vi "myVTOL Read-Write.vi"(5 "Fan Power Control (0V)":dbl(slide) scale=0.0..10.0, 7 "Control Mode (Manual)":bool, 8 "Error In":errorcluster, 9 "PID Settings":T1={"Proportional"=1.0, "Integral"=0.03, "Derivative"=0.05} {"Derivative" format="%.3f"; "Integral" format="%.2f"; "Proportional" format="%.3f"}, 10 "Set Point (2.1V)":dbl=2.1 step=0.01 format="%#_g V", 11 "task array in":refnum<k21>[](array[refnum])) -> (0 "Error Out":errorcluster, 1 "Sensor Reading":dbl=2.0424252344528213 format="%0.2f V", 2 "Fan Control Output [V]":dbl(knob)=5.428571428571428 scale=0.0..10.0, 3 "task array out":refnum<k21>[](array[refnum]), 4 "Waveform Chart":cluster{"data":dbl, "Set Point":dbl}(graph)={"data"=2.0424252344528213, "Set Point"=2.1})   [LabVIEW 2013]
uses:
  <vilib>/DAQmx/read.llb/DAQmx Read (Analog Wfm 1Chan NSamp).vi
  <vilib>/DAQmx/write.llb/DAQmx Write (Analog DBL 1Chan 1Samp).vi
  <vilib>/DAQmx/miscellaneous.llb/DAQmx Fill In Error Info.vi
panel:
  # "PID Gain Settings"
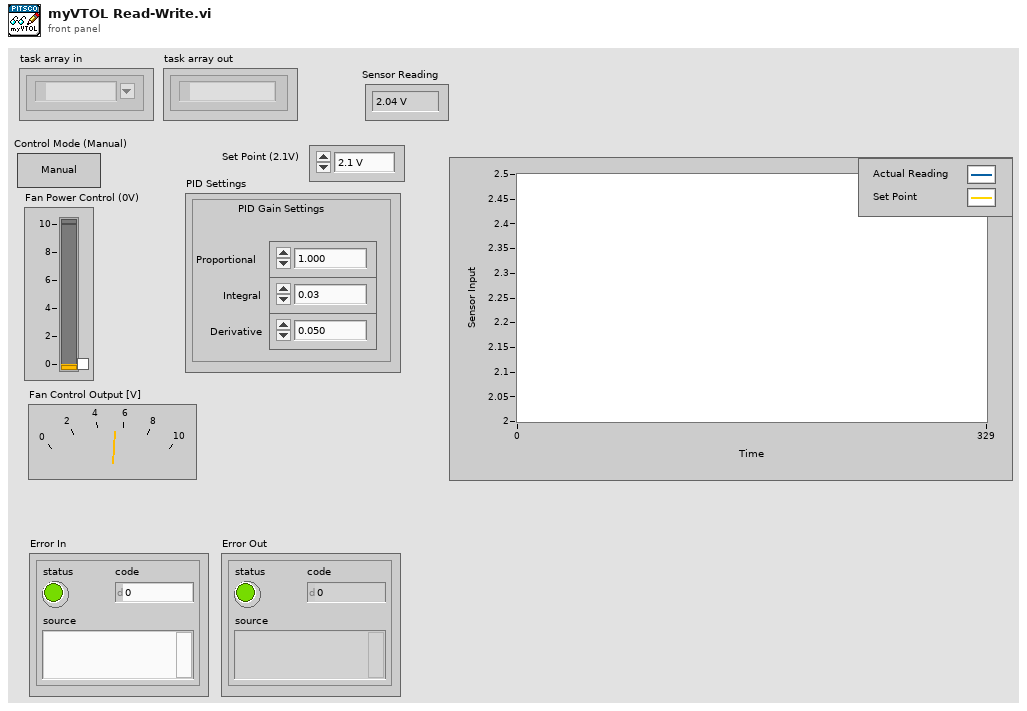
[diagram p1: front panel]
types:
  T1 = cluster{"Proportional":dbl, "Integral":dbl, "Derivative":dbl}
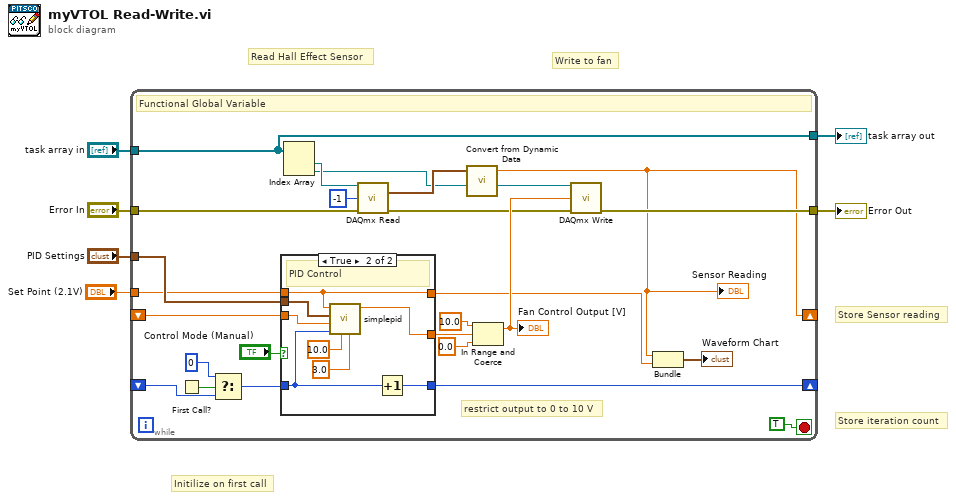
[diagram p0: block diagram]
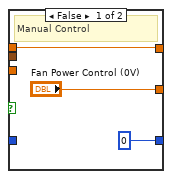
[diagram p2: hidden frame]
diagram:
  # "Initilize on first call"
  # "Write to fan"
  # "Read Hall Effect Sensor"
  # "Store Sensor reading"
  # "Store iteration count"
  n1 = while {
    tunnel: "Error In" -> [w31]
    tunnel: [w23] -> w2
    shift-right: [w13] -> _
    shift-left: _ -> [w25]
    shift-right: [w20] -> _
    shift-left: _ -> [w11]
    tunnel: "task array in" -> [w17]
    tunnel: [w17] -> w4
    tunnel: "PID Settings" -> [w15]
    tunnel: "Set Point (2.1V)" -> [w8]
    stop <- TRUE stop-if-true
    # "restrict output to 0 to 10 V"
    # "Functional Global Variable"
    n2 = First Call?() -> (First Call?: T/F=w12:bool)
    n3 = Select(t=0, s=w12, f=w11) -> (s? t:f=w9:i32)
    n4 = case shown="True" "Control Mode (Manual)" {
      tunnel: ["Fan Power Control (0V)" w42] -> w27
      tunnel: w25 -> [_ w37]
      tunnel: w9 -> [_ w38]
      tunnel: [0 ("output low") w39] -> w20
      tunnel: w15 -> [_ w36]
      tunnel: w8 -> [w32 w35]
      tunnel: [w32 w35] -> w7
      frame False {
        # "Manual Control"
      }
      frame True {
        # "PID Control"
        n5 = call "simplepid.vi"("minimum"=3.0 ("output low"), "maxim"=10.0 ("output high"), "Iteration"=w38, "pv"=w37, "PID Settings"=w36, "Target Sensor Reading"=w35) -> ("output variable"=w42:dbl)  [unwired: 5 in]
        n6 = Increment(x=w38) -> (x+1=w39:i32)
      }
    }
    n7 = Index Array(array=w17) -> (element #1=w19:refnum<k21>, element #2=w18:refnum<k21>)  [unwired: 2 in]
    n8 = call-poly <vilib>:"DAQmx Read.vi"("task/channels in"=w19, "number of samples per channel"=-1, "error in"=w31) -> ("data"=w21:waveform(dbl), "error out"=w24:errorcluster)  [unwired: 10 in, 1 out]
    n9 = call "Convert from Dynamic Data"("Dynamic Data Type"=w21) -> ("Scalar"=w13:dbl)  [unwired: 3 in]
    "Sensor Reading" <- w13
    n10 = In Range and Coerce(upper limit=10.0, x=w27, lower limit=0.0) -> (coerced(x)=w26:dbl)  [unwired: 1 out]
    "Fan Control Output [V]" <- w26
    n11 = call-poly <vilib>:"DAQmx Write.vi"("task/channels in"=w18, "data"=w26, "error in"=w24) -> ("error out"=w23:errorcluster)  [unwired: 10 in, 2 out]
    n12 = Bundle("Scalar"=w13, "Set Point (2.1V)"=w7) -> (→"Waveform Chart":cluster{"Scalar":dbl, "Set Point (2.1V)":dbl})  [unwired: 1 in]
  }
  "task array out" <- w4
  "Error Out" <- w2
